vi "Find Center.vi"(5 "Position":i32, 7 "Tray Number":dbl format="%#_13g", 8 "Assembly Type":string, 9 "XYZTheta":dbl[](array[numeric]), 10 "component thickness":dbl, 11 "Gantry In":refnum<k24>) -> (0 "Pedestal Heights":dbl[][](array[numeric]), 1 "XYZTheta Centers":dbl[][](array[numeric]), 3 "Gantry Out":refnum<k24>)   [LabVIEW 2021, in "Assembly Tray.lvclass"]
uses:
  Assembly Tray.lvclass
  Find Tray.ctl
  Controller/Camera/Machine Vision.ctl
  C:/Program Files (x86)/Aerotech/A3200/LabVIEW/2010/Bin/Aerotech.A3200.dll
  Program Files (x86)/Aerotech/A3200/LabVIEW/2010/Bin/Aerotech.A3200.dll
  Controller/Camera/Image processing.ctl
  Controller/Camera/Camera settings.ctl
  <vilib>/Utility/file.llb/Read Delimited Spreadsheet (DBL).vi
  Controller/Camera/Camera.lvclass
  Controller/Motion/A3200/A3200.lvclass
  Controller/Motion/Motion.lvclass
  <vilib>/vision/NI_Vision_Development_Module.lvlib
panel:
  out "Global Report.Standard Variation":sgl
  in  "BP check":bool
  out "Program Done?":bool
  out "Manual Mode?":bool
  in  "Enter Manual Mode":bool
  out "error out":errorcluster
  out "Radius (Real-World)":dbl
  out "Match found?":bool
  out "Distance as expected?":bool
  in  "Auto Submit":bool
  out "Instructions":string="Use the joystick to match the pattern recognition until a red circle appears.\nUse Z controls to focus if needed."
  out "resulting string":string
  out "Current Z High Speed":dbl
  out "Current XY High Speed":dbl
  out "current Z low speed":dbl
  out "current XY speed":dbl
  in  "Z high":dbl=12.5
  in  "XY high":dbl=50.0
  in  "Z low":dbl=0.05
  in  "XY low":dbl=0.1
  out "Low Speed":bool
  out "X":bool
  out "Y":bool
  out "Z":bool
  out "High Speed":bool
  out "Move by":dbl[](array[numeric])
  in  "Autofiducial (Beta)":bool
  out "maximum is best focus":dbl
  in  "Focus":bool
  in  "Camera settings":T1={"Gamma"=1.6, "Gain"=0, "Sharpness"=0, "Contrast"=0.0, "Exposure"=0.0078125} {"Exposure" min=0.000244140625 max=0.5 scale=0.0002..0.5; "Contrast" min=0.0 max=1.0 scale=0.001..1.0; "Sharpness" min=0 max=2 step=1 scale=0.0..2.0; "Gain" min=0 max=100 step=1 scale=0.1..100.0; "Gamma" min=0.01 max=10.0 scale=0.01..10.0}
  in  "Image processing":T2={"Brightness"=128.0, "Contrast"=45.0, "Gamma"=1.0471123} {"Brightness" scale=0.0..400.0; "Contrast" scale=0.0..90.0; "Gamma" scale=0.005..5.0}
  in  "Override camera presets":bool
  out "Both fiducials recorded":bool
  in  "Machine Vision":T3
  out "Right Fiducial":dbl[](array[numeric]) format="%.6g"
  out "Left Fiducial":dbl[](array[numeric]) format="%.6g"
  out "Gantry":dbl[](array[numeric]) format="%.6g"
  out "Sum":dbl[](array[numeric]) format="%.6g"
  out "Camera":dbl[](array[numeric]) format="%.6g"
  in  "Carrier Tray":T4
  out "Image":T5(plugin-control)
  out "Center":dbl[](array[numeric]) format="%.6g"
  in  "Position Number":i16=1
  in  "Go to Center":bool
  in  "Calculate":bool
  in  "Record Top Right":bool
  in  "Record Top Left":bool
  in  "Go to Top Right Fiducial":bool
  in  "Go to Top Left Fiducial":bool
  in  "Joystick":bool
  in  "Stop":bool
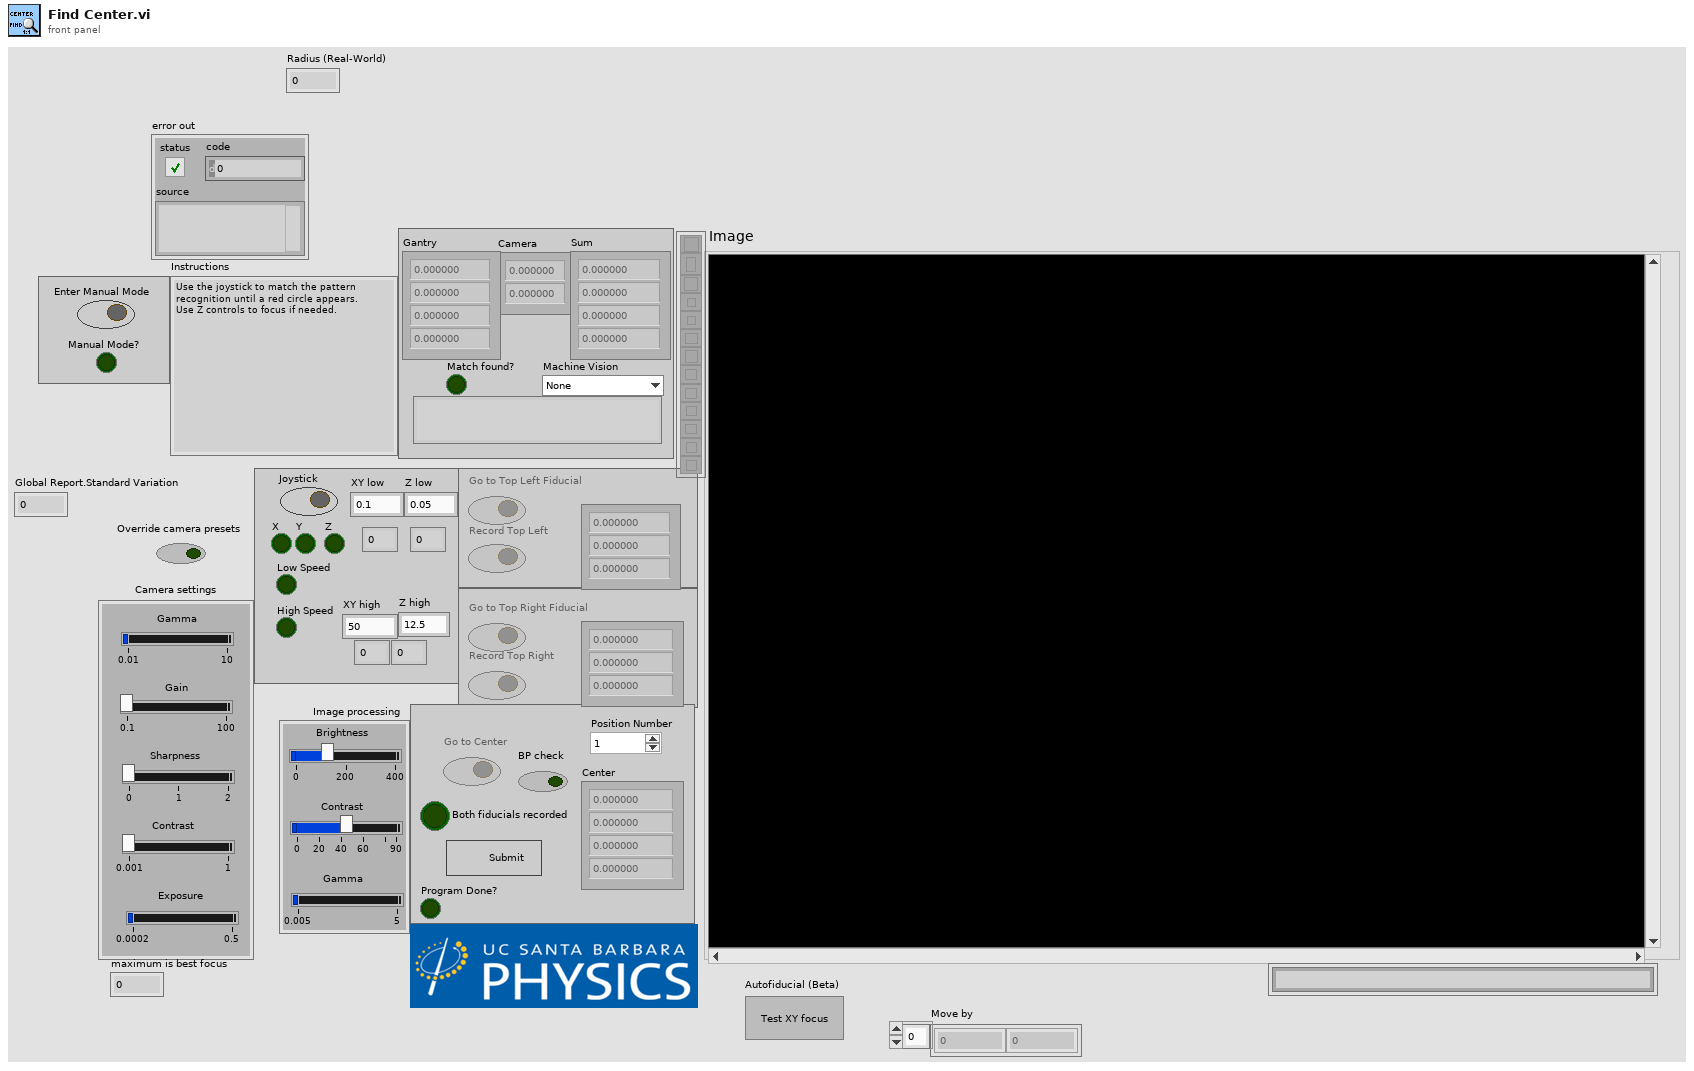
[diagram p1: front panel]
types:
  T1 = typedef "Camera.lvclass/Camera settings.ctl" = cluster{"Gamma":dbl, "Gain":i64, "Sharpness":i64, "Contrast":dbl, "Exposure":dbl}
  T2 = typedef "Camera.lvclass/Image processing.ctl" = cluster{"Brightness":sgl, "Contrast":sgl, "Gamma":sgl}
  T3 = typedef "Camera.lvclass/Machine Vision.ctl" = enum16{"None", "Assembly Tray Circle", "Assembly Tray Fiducial", "Partial Hexaboard", "sensor edge init", "HB edge init", "sensor edge pos1", "sensor edge pos2", "HB edge pos1", "HB edge pos2", "Sensor CH1-2", "HB CH1", "HB CH2", "V3 Sensor Circle", "Hexaboard Circle", "sensor CH1 check", "HB CH1 check ", "sensor ID"}
  T4 = typedef "Assembly Tray.lvclass/Find Tray.ctl" = cluster{"Gantry Fiducials":dbl[], "Relative Coordinates":dbl[][], "Camera Fiducials":dbl[][], "XYZTheta Centers":dbl[][], "Workspace Center":dbl[], "Syringe Relative Coordinates":dbl[], "Gantry Region":dbl, "Fiducials":path, "New Fiducials":dbl[][], "Past Fiducials":dbl[][], "XYZTheta":dbl[], "Pedestal Heights":dbl[][], "Assembly Type":string, "Tray Number":string, "Position":i32, "Protomodule?":bool, "avg value count":dbl[], "Previous Avgs":dbl[][], "Offset pins":dbl[][]}
  T5 = typedef "IMAQ Image.ctl" = refnum<image>
  T6 = cluster{"Average Strength":dbl, "Radius (Real-World)":dbl, "Match found?":bool, "initial angle":sgl, "Global Report":cluster{"Mean Value":sgl, "Standard Variation":sgl, "Minimal Value":sgl, "Maximal Value":sgl, "Area (calibrated)":sgl, "Area (pixels)":u32, "%":sgl, "Calibration Valid":bool}}
  T7 = enum8{"Enabled", "Disabled", "Disabled and Grayed Out"}
  T8 = typedef "File Paths.ctl" = cluster{"Glue Pattern Folder":path, "Carrier Tray Folder":path, "Pick Up Tool Fixture Folder":path, "Components Folder":path, "Bellows Tool Offset.txt":path, "Pick Up Tool Offset.txt":path, "Dispense Tip Offset.txt":path, "Log Files":path, "Gantry Assembly Map.txt":path, "Syringe and offset map.txt":path, "Controllers Folder":path, "Local dbase config":path}
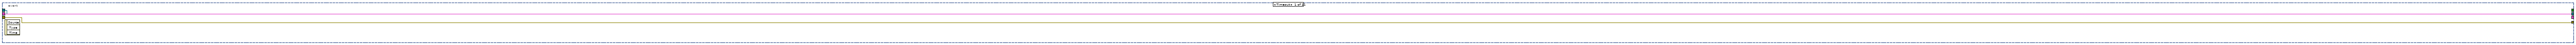
[diagram p3: hidden frame]
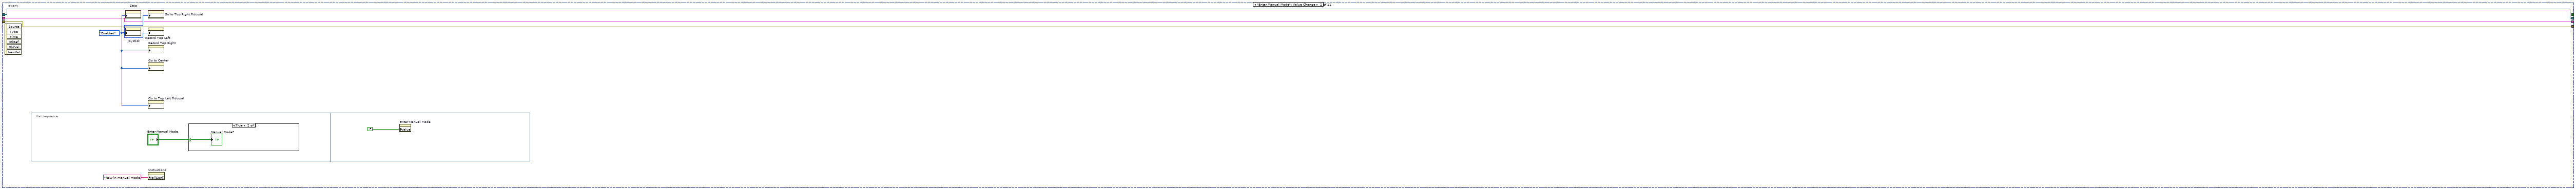
[diagram p4: hidden frame]
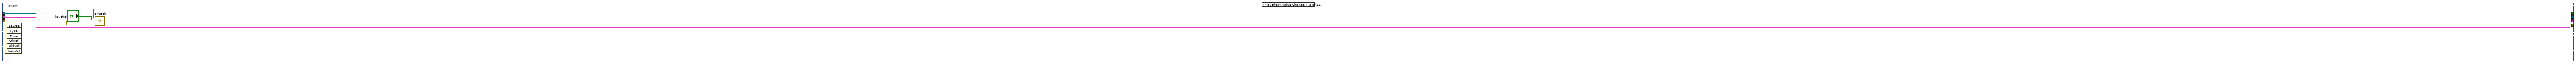
[diagram p6: hidden frame]
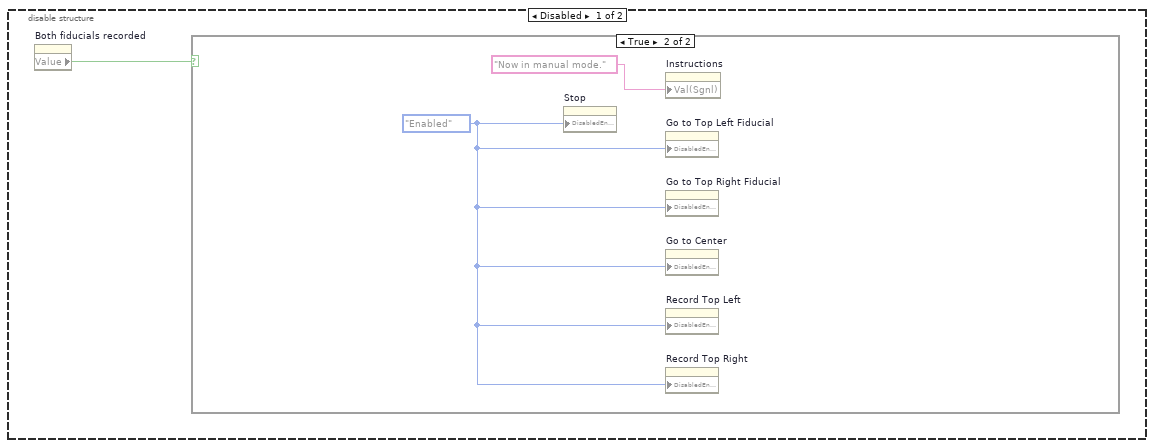
[diagram p7: hidden frame]
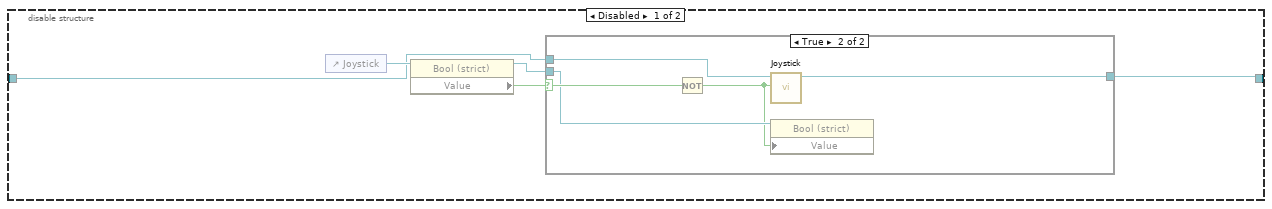
[diagram p9: hidden frame]
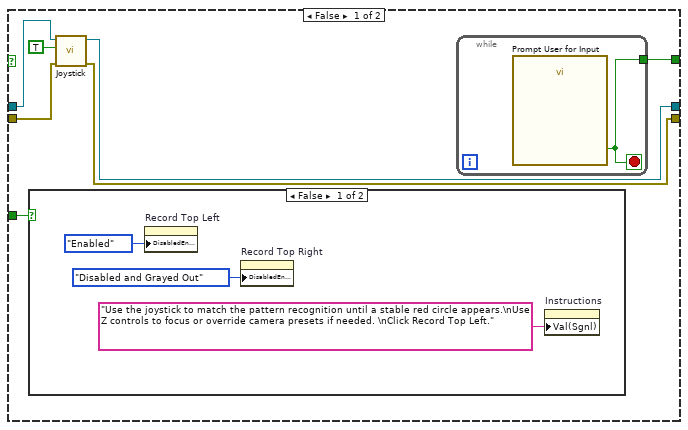
[diagram p12: hidden frame]
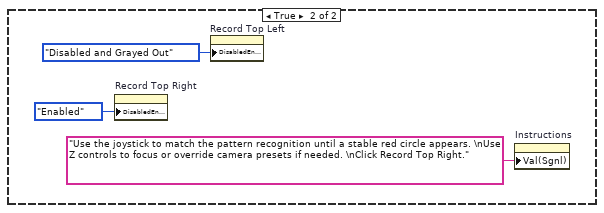
[diagram p13: hidden frame]
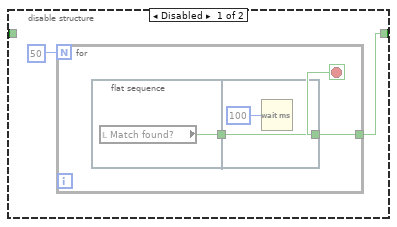
[diagram p19: hidden frame]
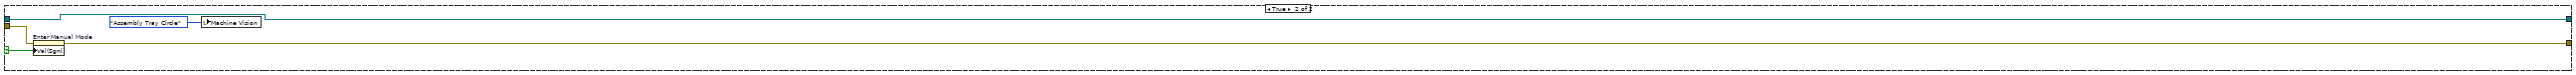
[diagram p20: hidden frame]
diagram:
  n1 = flat-sequence {
    tunnel: [w17] -> w9
    tunnel: ["Gantry In"] -> w8
    tunnel: [w16] -> w7
    tunnel: [w14] -> w4
    tunnel: [w29] -> w5
    tunnel: w9 -> [w29]
    tunnel: [w27] -> w2
    tunnel: w8 -> [w27]
    tunnel: w7 -> [w26]
    tunnel: [w26] -> w6
    tunnel: [w25] -> w1
    tunnel: w4 -> [w24]
    frame #0 {
      n2 = Decrement(x="Position") -> (x-1=w21:i32)
      n3 = call "Find Center Setup.vi"("XYZTheta"="XYZTheta", "Assembly Type"="Assembly Type", "Position"=w21, "Tray Number"="Tray Number", "Carrier Tray"="Carrier Tray") -> ("Assembly Tray Out"=w17:T4)  [unwired: 6 in]
      n4 = call "Get Camera Object.vi"() -> ("error out"=w14:errorcluster, "Camera out"=w16:refnum<class "Camera.lvclass">)  [unwired: 10 in]
    }
    frame #1 {
      n5 = control-ref of="This VI"() -> (w28:refnum<vi>)
      n6 = invoke class="VI" method="Default Vals.Reinit All"(reference=w28, error in=w24) -> (error out=w25:errorcluster)  [unwired: 1 in, 2 out]
    }
  }
  n7 = while {
    shift-right: [w36] -> _
    shift-left: w6 -> [w37]
    tunnel: w2 -> [w34]
    shift-right: [w33] -> _
    shift-left: _ -> [_]
    shift-right: [w31] -> _
    shift-left: w1 -> [w32]
    i -> [w35]
    stop <- w30 stop-if-true
    n8 = flat-sequence {
      tunnel: [w58] -> w36
      tunnel: w34 -> [w44]
      tunnel: [w43] -> w33
      tunnel: w32 -> [w42]
      tunnel: [w41] -> w31
      tunnel: w37 -> [w61]
      tunnel: w35 -> [w56]
      tunnel: [w39] -> w30
      frame #0 {
        n9 = in-place {
          in-place-border: w44 -> [w88]
          in-place-border: [w69] -> w47
          in-place-border: w42 -> [w64]
          in-place-border: [w62] -> w48
          # "Joystck Status"
          n10 = call "Get Joytick Status.vi"("error in (no error)"=w64, "Gantry In"=w88) -> ("error out"=w63:errorcluster, "JoystickLowSpeedActive"=w82:bool, "Joystick Status"=w84:bool[], "Gantry Out"=w70:refnum<k24>, "High Speeds"=w66:dbl[], "Low Speeds"=w65:dbl[])  [unwired: 4 in]
          n11 = Build Array("XY low", "XY low", "XY low", "Z low") -> (w68:dbl[])
          n12 = Build Array("XY high", "XY high", "XY high", "Z high") -> (w67:dbl[])
          n13 = call "Set Joystick Speed.vi"("error in (no error)"=w63, "High Speed Inputs"=w67, "Low Speed Inputs"=w68, "Gantry"=w70) -> ("error out"=w62:errorcluster, "Controller Out"=w69:refnum<k24>)  [unwired: 6 in]
          n14 = Or Array Elements(Boolean array=w84) -> (logical OR=w80:bool)
          n15 = Not(x=w82) -> (.not. x?=w81:bool)
          n16 = Index Array(array=w66) -> (element #1=→"Current XY High Speed":dbl, element #3=→"Current Z High Speed":dbl)  [unwired: 3 in, 1 out]
          n17 = Index Array(array=w65) -> (element #1=→"current XY speed":dbl, element #3=→"current Z low speed":dbl)  [unwired: 3 in, 1 out]
          n18 = Index Array(array=w84) -> (element #1=→"X":bool, element #2=→"Y":bool, element #3=→"Z":bool)  [unwired: 3 in]
          n19 = And(x=w80, y=w82) -> (x .and. y?=→"Low Speed":bool)
          n20 = And(x=w81, y=w80) -> (x .and. y?=→"High Speed":bool)
        }
        n21 = Equal To 0?(x=w56) -> (x = 0?=w55:bool)
        n22 = local read "Program Done?"() -> (w39:bool)
        n23 = call "Camera.vi"("Camera in"=w61, "Stop"=w39, "BCG Image Processing"="Image processing", "Machine Vision"="Machine Vision", "Camera settings"="Camera settings", "Loop 0"=w55, "Override presets"="Override camera presets") -> ("Camera out"=w58:refnum<class "Camera.lvclass">, "output cluster"=w54:T6, "Image"=→"Image":T5, "Camera"=w40:dbl[])  [unwired: 5 in, 4 out]
        "Camera" <- w40
        n24 = call "Get Current Position.vi"("error in (no error)"=w48, "Gantry In"=w47) -> ("error out"=w41:errorcluster, "XYZTheta Out"=w46:dbl[], "Gantry Out"=w43:refnum<k24>)  [unwired: 7 in]
        "Gantry" <- w46
        n25 = Unbundle By Name(w54) -> ("Average Strength"=→"maximum is best focus":dbl, "Radius (Real-World)"=→"Radius (Real-World)":dbl, "Match found?"=→"Match found?":bool, "Global Report.Standard Variation"=w38:sgl)
        "Global Report.Standard Variation" <- w38
        n26 = shared-variable ".\\Assembly Tray.lvclass\\BP Standard Variation"(w38) -> ()  [unwired: 1 in, 1 out]
        n27 = Add(x=w46, y=w40) -> (x+y=→"Sum":dbl[])
      }
    }
  }
  n28 = while {
    shift-right: [w98] -> w13
    shift-left: w5 -> [w99]
    shift-right: [w95] -> w11
    shift-left: w2 -> [w96]
    tunnel: w5 -> [w91]
    shift-right: [w89] -> w3
    shift-left: w1 -> [w90]
    i -> [w94]
    stop <- w97 stop-if-true
    n29 = event shown="[3] \"Go to Top Left Fiducial\", \"Go to Top Right Fiducial\": Value Change" {
      selector: _ -> [_ _ _ _ _ _ _ _ _ _ _]
      dyn-events: _ -> [_ _ _ _ _ _ _ _ _ _ _]
      timeout: _ -> [_ _ _ _ _ _ _ _ _ _ _]
      tunnel: [w111 w114 w125 w143 w366 w425 w563 w759 w837 w857 w930] -> w98
      tunnel: w99 -> [w111 w114 w125 w143 w362 w425 w564 w759 w838 w857 w930]
      tunnel: [_ _ _ _ _ _ _ _ _ w858 _] -> w97
      tunnel: w96 -> [w110 w115 w124 w142 w361 w424 w569 w769 w835 w861 w932]
      tunnel: [w110 w115 w122 w141 w360 w423 w569 w762 w832 w860 w933] -> w95
      tunnel: [w109 w113 w120 w132 w355 w419 w557 w763 w829 w865 w928] -> w89
      tunnel: w90 -> [w109 w113 w121 w133 w357 w418 w560 w768 w829 w862 w929]
      event Timeout {
        n30 = event-data() -> ()  [unwired: 1 in, 3 out]
      }
      event "Enter Manual Mode": Value Change {
        w116 = T7."Enabled" ("Disabled")
        n31 = event-data() -> ()  [unwired: 1 in, 6 out]
        n32 = flat-sequence {
          frame #0 {
            n33 = case shown="True" "Enter Manual Mode" {
              selector: "Enter Manual Mode" -> [_ w118]
              frame False {
              }
              frame True {
                "Manual Mode?" <- w118
              }
            }
          }
          frame #1 {
            n34 = property on="Enter Manual Mode" class="Bool (strict)"("Value"=FALSE ("Enter Manual Mode")) -> ()  [unwired: 2 in, 2 out]
          }
        }
        n35 = property on="Stop" class="Bool"("DisabledEnum"=w116) -> ()  [unwired: 2 in, 2 out]
        n36 = property on="Joystick" class="Bool (strict)"("DisabledEnum"=w116) -> ()  [unwired: 2 in, 2 out]
        n37 = property on="Go to Top Right Fiducial" class="Bool (strict)"("DisabledEnum"=w116) -> ()  [unwired: 2 in, 2 out]
        n38 = property on="Record Top Left" class="Bool (strict)"("DisabledEnum"=w116) -> ()  [unwired: 2 in, 2 out]
        n39 = property on="Record Top Right" class="Bool (strict)"("DisabledEnum"=w116) -> ()  [unwired: 2 in, 2 out]
        n40 = property on="Go to Center" class="Bool"("DisabledEnum"=w116) -> ()  [unwired: 2 in, 2 out]
        n41 = property on="Go to Top Left Fiducial" class="Bool (strict)"("DisabledEnum"=w116) -> ()  [unwired: 2 in, 2 out]
        n42 = property on="Instructions" class="Str"("Val(Sgnl)"="Now in manual mode." ("Value (Signaling)")) -> ()  [unwired: 2 in, 2 out]
      }
      event "Joystick": Value Change {
        n43 = event-data() -> ()  [unwired: 1 in, 6 out]
        n44 = call "Joystick.vi"("error in (no error)"=w121, "Joystick"="Joystick", "Gantry In"=w124) -> ("error out"=w120:errorcluster, "Gantry Out"=w122:refnum<k24>)  [unwired: 7 in]
      }
      event "Go to Top Left Fiducial", "Go to Top Right Fiducial": Value Change {
        n45 = event-data() -> ()  [unwired: 1 in, 6 out]
        n46 = disable-structure shown="Enabled" {
          frame Disabled {
            n47 = property on="Both fiducials recorded" class="Bool (strict)"() -> ("Value"=w144:bool)  [unwired: 2 in, 2 out]
            n48 = case shown="True" w144 {
              frame False {
              }
              frame True {
                w145 = T7."Enabled" ("Disabled")
                n49 = property on="Stop" class="Bool"("DisabledEnum"=w145) -> ()  [unwired: 2 in, 2 out]
                n50 = property on="Instructions" class="Str"("Val(Sgnl)"="Now in manual mode." ("Value (Signaling)")) -> ()  [unwired: 2 in, 2 out]
                n51 = property on="Go to Top Left Fiducial" class="Bool (strict)"("DisabledEnum"=w145) -> ()  [unwired: 2 in, 2 out]
                n52 = property on="Go to Top Right Fiducial" class="Bool (strict)"("DisabledEnum"=w145) -> ()  [unwired: 2 in, 2 out]
                n53 = property on="Go to Center" class="Bool"("DisabledEnum"=w145) -> ()  [unwired: 2 in, 2 out]
                n54 = property on="Record Top Left" class="Bool (strict)"("DisabledEnum"=w145) -> ()  [unwired: 2 in, 2 out]
                n55 = property on="Record Top Right" class="Bool (strict)"("DisabledEnum"=w145) -> ()  [unwired: 2 in, 2 out]
              }
            }
          }
          frame Enabled {
          }
        }
        n56 = disable-structure shown="Enabled" {
          disable-tunnel: w142 -> [w149 w158]
          disable-tunnel: [w147 w158] -> w140
          frame Disabled {
            n57 = control-ref of="Joystick"() -> (w151:refnum<vi>)
            n58 = property class="Bool (strict)"(reference=w151) -> (reference out=w148:refnum<vi>, "Value"=w150:bool)  [unwired: 1 in, 1 out]
            n59 = case shown="True" w150 {
              selector: w150 -> [_ w157]
              tunnel: w149 -> [w152 w155]
              tunnel: [w152 w154] -> w147
              tunnel: w148 -> [_ w156]
              frame False {
              }
              frame True {
                n60 = Not(x=w157) -> (.not. x?=w153:bool)
                n61 = call "Joystick.vi"("Joystick"=w153, "Gantry In"=w155) -> ("Gantry Out"=w154:refnum<k24>)  [unwired: 8 in, 1 out]
                n62 = property class="Bool (strict)"(reference=w156, "Value"=w153) -> ()  [unwired: 1 in, 2 out]
              }
            }
          }
          frame Enabled {
          }
        }
        n63 = Unbundle By Name "Unbundle By Name"(w143) -> ("Gantry Fiducials"=w135:dbl[])
        n64 = flat-sequence {
          tunnel: w135 -> [w160]
          tunnel: w140 -> [w161]
          tunnel: [w161] -> w131
          tunnel: [w160] -> w129
          tunnel: ["Go to Top Right Fiducial"] -> w127
          tunnel: ["Go to Top Right Fiducial"] -> w134
          tunnel: w131 -> [w165]
          tunnel: [w165] -> w130
          tunnel: w129 -> [w164]
          tunnel: [w164] -> w128
          tunnel: w127 -> [w163]
          tunnel: [w163] -> w126
          tunnel: [w183] -> w139
          tunnel: [w179] -> w136
          tunnel: w130 -> [w177]
          tunnel: w128 -> [w174]
          tunnel: w126 -> [w171]
          tunnel: w133 -> [w167]
          tunnel: w139 -> [w185]
          tunnel: [w185] -> w138
          tunnel: [w184] -> w137
          tunnel: w136 -> [w184]
          tunnel: [w188] -> w141
          tunnel: [w187] -> w132
          tunnel: w137 -> [w190]
          tunnel: w134 -> [w191]
          tunnel: w138 -> [w192]
          frame #0 {
          }
          frame #1 {
            w162 = FALSE ("Go to Top Right Fiducial")
            n65 = property on="Go to Top Left Fiducial" class="Bool (strict)"("Value"=w162) -> ()  [unwired: 2 in, 2 out]
            n66 = property on="Go to Top Right Fiducial" class="Bool (strict)"("Value"=w162) -> ()  [unwired: 2 in, 2 out]
          }
          frame #2 {
            w180 = T7."Disabled and Grayed Out" ("Disabled")
            n67 = Select(t=3, s=w171, f=0) -> (s? t:f=w169:i32)
            n68 = call "Joystick.vi"("error in (no error)"=w167, "Joystick"=FALSE, "Gantry In"=w177) -> ("error out"=w175:errorcluster, "Gantry Out"=w178:refnum<k24>)  [unwired: 7 in]
            n69 = Array Subset "Array Subset"(array=w174, index=w169, length=3) -> (w173:dbl[])
            n70 = property on="Instructions" class="Str"("Val(Sgnl)"="Wait for movement to stop." ("Value (Signaling)")) -> ()  [unwired: 2 in, 2 out]
            n71 = property on="Go to Center" class="Bool"("DisabledEnum"=w180) -> ()  [unwired: 2 in, 2 out]
            n72 = property on="Stop" class="Bool"("DisabledEnum"=w180) -> ()  [unwired: 2 in, 2 out]
            n73 = property on="Record Top Right" class="Bool (strict)"("DisabledEnum"=w180) -> ()  [unwired: 2 in, 2 out]
            n74 = property on="Go to Top Right Fiducial" class="Bool (strict)"("DisabledEnum"=w180) -> ()  [unwired: 2 in, 2 out]
            n75 = property on="Go to Top Left Fiducial" class="Bool (strict)"("DisabledEnum"=w180) -> ()  [unwired: 2 in, 2 out]
            n76 = property on="Record Top Left" class="Bool (strict)"("DisabledEnum"=w180) -> ()  [unwired: 2 in, 2 out]
            n77 = local write "Machine Vision"(Machine_Vision."Assembly Tray Fiducial" ("Machine Vision")) -> ()
            n78 = call "ClearXYZTheta Go.vi"("error in (no error)"=w175, "Speed"=300.0, "XYZTheta In"=w173, "Gantry In"=w178) -> ("error out"=w179:errorcluster, "Gantry Out"=w183:refnum<k24>)  [unwired: 5 in, 1 out]
          }
          frame #3 {
            n79 = disable-structure shown="Enabled" {
              frame Enabled {
                n80 = Wait (ms)(milliseconds to wait=u32 1000) -> ()  [unwired: 1 out]
              }
              frame Disabled {
              }
            }
          }
          frame #4 {
            n81 = local read "Manual Mode?"() -> (w189:bool)
            n82 = case shown="False" w189 {
              selector: w189 -> [_ w352]
              tunnel: w192 -> [w214 w353]
              tunnel: [w194 w353] -> w188
              tunnel: w191 -> [w195 _]
              tunnel: w190 -> [w213 w351]
              tunnel: [w193 w350] -> w187
              frame False {
                n83 = flat-sequence {
                  tunnel: w214 -> [w239]
                  tunnel: w213 -> [w237]
                  tunnel: [w238] -> w212
                  tunnel: [w236] -> w211
                  tunnel: [w235] -> w210
                  tunnel: [w234] -> w209
                  tunnel: w212 -> [w299]
                  tunnel: w211 -> [w298]
                  tunnel: w210 -> [w297]
                  tunnel: w209 -> [w296]
                  tunnel: [w299] -> w208
                  tunnel: [w298] -> w206
                  tunnel: [w297] -> w204
                  tunnel: [w296] -> w202
                  tunnel: w208 -> [w303]
                  tunnel: [w303] -> w207
                  tunnel: w206 -> [w302]
                  tunnel: [w302] -> w205
                  tunnel: w204 -> [w301]
                  tunnel: [w301] -> w203
                  tunnel: w202 -> [w300]
                  tunnel: [w300] -> w201
                  tunnel: w207 -> [w311]
                  tunnel: w205 -> [w310]
                  tunnel: w203 -> [w306]
                  tunnel: w201 -> [w309]
                  tunnel: [w308] -> w199
                  tunnel: [w307] -> w200
                  tunnel: [w305] -> w196
                  frame #0 {
                    n84 = for {
                      N: 50 -> [_]
                      tunnel: [w242] -> w240
                      tunnel: [w241] -> w232
                      stop <- w242 stop-if-true
                      n85 = flat-sequence {
                        tunnel: [w245] -> w243
                        tunnel: [w244] -> w241
                        tunnel: [w247] -> w242
                        tunnel: w243 -> [w247]
                        frame #0 {
                          n86 = local read "Match found?"() -> (w245:bool)
                          n87 = local read "Camera"() -> (w244:dbl[])
                        }
                        frame #1 {
                          n88 = Wait (ms)(milliseconds to wait=u32 100) -> ()  [unwired: 1 out]
                        }
                      }
                    }
                    n89 = case shown="False" w240 {
                      selector: w240 -> [_ w292]
                      tunnel: w239 -> [w251 w294]
                      tunnel: [w253 w294] -> w238
                      tunnel: w237 -> [w250 w293]
                      tunnel: [w252 w293] -> w236
                      tunnel: [w249 w292] -> w235
                      tunnel: [w248 w291] -> w234
                      tunnel: w232 -> [_ w291]
                      frame False {
                        n90 = flat-sequence {
                          tunnel: [w265] -> w253
                          tunnel: [w264] -> w252
                          tunnel: w251 -> [w263]
                          tunnel: w250 -> [w262]
                          tunnel: [w257] -> w249
                          tunnel: [w254] -> w248
                          frame #0 {
                            n91 = call "Base File Path.vi"() -> ("Paths Out"=w259:T8)  [unwired: 11 in]
                            n92 = Unbundle By Name(w259) -> ("Controllers Folder"=w260:path)
                            n93 = String To Path(string="Scan.txt") -> (path=w261:path)
                            n94 = Build Path(base path=w260, name or relative path=w261) -> (appended path=w256:path)
                            n95 = call-poly <vilib>:"Read Delimited Spreadsheet.vi"("file path (dialog if empty)"=w256) -> ("all rows"=w255:dbl[][])  [unwired: 9 in, 5 out]
                            n96 = for {
                              shift-right: [w275] -> w265
                              shift-left: w263 -> [w276]
                              tunnel: w255 -> [w274] mode=indexing
                              shift-right: [w272] -> w264
                              shift-left: w262 -> [w273]
                              tunnel: [w267] -> w257
                              tunnel: [w266] -> w254
                              stop <- w267 stop-if-true
                              n97 = flat-sequence {
                                tunnel: w276 -> [w283]
                                tunnel: w274 -> [w281]
                                tunnel: w273 -> [w279]
                                tunnel: [w282] -> w271
                                tunnel: [w278] -> w270
                                tunnel: w271 -> [w284]
                                tunnel: w270 -> [w285]
                                tunnel: [w284] -> w269
                                tunnel: [w285] -> w268
                                tunnel: [w289] -> w272
                                tunnel: [w290] -> w275
                                tunnel: w269 -> [w290]
                                tunnel: w268 -> [w289]
                                tunnel: [w288] -> w267
                                tunnel: [w287] -> w266
                                frame #0 {
                                n98 = call "XY Go.vi"("Increment?"=TRUE, "error in (no error)"=w279, "Speed"=0.1, "XY In"=w281, "Gantry In"=w283) -> ("error out"=w278:errorcluster, "Gantry Out"=w282:refnum<k24>)  [unwired: 4 in, 1 out]
                                }
                                frame #1 {
                                n99 = disable-structure shown="Enabled" {
                                disable-tunnel: w284 -> [_ _]
                                frame Enabled {
                                n100 = Wait (ms)(milliseconds to wait=u32 500) -> ()  [unwired: 1 out]
                                }
                                frame Disabled {
                                }
                                }
                                }
                                frame #2 {
                                n101 = local read "Match found?"() -> (w288:bool)
                                n102 = local read "Camera"() -> (w287:dbl[])
                                }
                              }
                            }
                          }
                        }
                      }
                      frame True {
                      }
                    }
                  }
                  frame #1 {
                    n103 = local write "Machine Vision"(Machine_Vision."Assembly Tray Circle" ("Machine Vision")) -> ()
                  }
                  frame #2 {
                    n104 = disable-structure shown="Enabled" {
                      frame Enabled {
                        n105 = Wait (ms)(milliseconds to wait=u32 1000) -> ()  [unwired: 1 out]
                      }
                      frame Disabled {
                      }
                    }
                  }
                  frame #3 {
                    n106 = case shown="True" w306 {
                      selector: w306 -> [w312 w315]
                      tunnel: w311 -> [w314 w325]
                      tunnel: [w314 w324] -> w308
                      tunnel: w310 -> [w313 w323]
                      tunnel: [w313 w322] -> w307
                      tunnel: w309 -> [_ w321]
                      tunnel: [w312 w316] -> w305
                      frame False {
                      }
                      frame True {
                        n107 = flat-sequence {
                          tunnel: w325 -> [w333]
                          tunnel: w323 -> [w331]
                          tunnel: w321 -> [w326]
                          tunnel: [w332] -> w320
                          tunnel: [w330] -> w319
                          tunnel: w320 -> [w335]
                          tunnel: w319 -> [w334]
                          tunnel: [w335] -> w318
                          tunnel: [w334] -> w317
                          tunnel: [w339] -> w322
                          tunnel: [w340] -> w324
                          tunnel: w318 -> [w340]
                          tunnel: w317 -> [w339]
                          tunnel: [w338] -> w316
                          tunnel: w315 -> [w337]
                          frame #0 {
                            n108 = call "XY Go.vi"("Increment?"=TRUE, "error in (no error)"=w331, "Speed"=5.0, "XY In"=w326, "Gantry In"=w333) -> ("error out"=w330:errorcluster, "Gantry Out"=w332:refnum<k24>)  [unwired: 4 in, 1 out]
                            n109 = property on="Instructions" class="Str"("Val(Sgnl)"="Fiducial found." ("Value (Signaling)")) -> ()  [unwired: 2 in, 2 out]
                          }
                          frame #1 {
                            n110 = disable-structure shown="Enabled" {
                              frame Enabled {
                                n111 = Wait (ms)(milliseconds to wait=u32 1000) -> ()  [unwired: 1 out]
                              }
                              frame Disabled {
                              }
                            }
                          }
                          frame #2 {
                            n112 = disable-structure shown="Enabled" {
                              disable-tunnel: [w342 w348] -> w338
                              disable-tunnel: w337 -> [_ w348]
                              frame Disabled {
                                n113 = for {
                                N: 50 -> [_]
                                tunnel: [w343] -> w342
                                stop <- w343 stop-if-true
                                n114 = flat-sequence {
                                tunnel: [w345] -> w344
                                tunnel: [w347] -> w343
                                tunnel: w344 -> [w347]
                                frame #0 {
                                n115 = local read "Match found?"() -> (w345:bool)
                                }
                                frame #1 {
                                n116 = Wait (ms)(milliseconds to wait=u32 100) -> ()  [unwired: 1 out]
                                }
                                }
                                }
                              }
                              frame Enabled {
                              }
                            }
                          }
                        }
                      }
                    }
                  }
                }
                n117 = case shown="True" w196 {
                  selector: w196 -> [_ w231]
                  tunnel: [w216 w231] -> w198
                  tunnel: w199 -> [w220 w230]
                  tunnel: [w219 w230] -> w194
                  tunnel: w200 -> [w218 w229]
                  tunnel: [w217 w229] -> w197
                  tunnel: w195 -> [w215 _]
                  frame False {
                    n118 = case shown="False" w215 {
                      frame False {
                        n119 = property on="Record Top Left" class="Bool (strict)"("DisabledEnum"=T7."Enabled" ("Disabled")) -> ()  [unwired: 2 in, 2 out]
                        n120 = property on="Record Top Right" class="Bool (strict)"("DisabledEnum"=T7."Disabled and Grayed Out" ("Disabled")) -> ()  [unwired: 2 in, 2 out]
                        n121 = property on="Instructions" class="Str"("Val(Sgnl)"="Use the joystick to match the pattern recognition until a stable red circle appears.\nUse Z controls to focus or override camera presets if needed. \nClick Record Top Left.") -> ()  [unwired: 2 in, 2 out]
                      }
                      frame True {
                        n122 = property on="Record Top Right" class="Bool (strict)"("DisabledEnum"=T7."Enabled" ("Disabled")) -> ()  [unwired: 2 in, 2 out]
                        n123 = property on="Record Top Left" class="Bool (strict)"("DisabledEnum"=T7."Disabled and Grayed Out" ("Disabled")) -> ()  [unwired: 2 in, 2 out]
                        n124 = property on="Instructions" class="Str"("Val(Sgnl)"="Use the joystick to match the pattern recognition until a stable red circle appears. \nUse Z controls to focus or override camera presets if needed. \nClick Record Top Right.") -> ()  [unwired: 2 in, 2 out]
                      }
                    }
                    n125 = call "Joystick.vi"("error in (no error)"=w218, "Joystick"=TRUE, "Gantry In"=w220) -> ("error out"=w217:errorcluster, "Gantry Out"=w219:refnum<k24>)  [unwired: 7 in]
                    n126 = while {
                      tunnel: [w222] -> w216
                      stop <- w222 stop-if-true
                      n127 = call "Prompt User for Input"() -> ("Target line up?"=w222:bool)  [unwired: 17 in, 2 out]
                    }
                  }
                  frame True {
                  }
                }
                n128 = property on="Focus" class="Bool (strict)"(error in=w197, "Val(Sgnl)"=w198) -> (error out=w193:errorcluster)  [unwired: 1 in, 1 out]
              }
              frame True {
                n129 = property on="Enter Manual Mode" class="Bool (strict)"(error in=w351, "Val(Sgnl)"=w352) -> (error out=w350:errorcluster)  [unwired: 1 in, 1 out]
                n130 = local write "Machine Vision"(Machine_Vision."Assembly Tray Circle" ("Machine Vision")) -> ()
              }
            }
          }
        }
      }
      event "Record Top Left", "Record Top Right": Value Change {
        n131 = event-data() -> ()  [unwired: 1 in, 6 out]
        n132 = flat-sequence {
          tunnel: ["Record Top Right"] -> w354
          frame #0 {
          }
          frame #1 {
            w368 = FALSE ("Record Top Left")
            n133 = property on="Record Top Left" class="Bool (strict)"("Value"=w368) -> ()  [unwired: 2 in, 2 out]
            n134 = property on="Record Top Right" class="Bool (strict)"("Value"=w368) -> ()  [unwired: 2 in, 2 out]
          }
        }
        n135 = Boolean To (0,1)(Boolean=w354) -> (0, 1=w363:i16)
        n136 = in-place {
          in-place-border: [w387] -> w364
          in-place-border: w363 -> [w380]
          in-place-border: w361 -> [w382]
          in-place-border: [w381] -> w360
          in-place-border: w357 -> [w375]
          in-place-border: [w373] -> w356
          n137 = in-place-cluster #1(w362) -> ("Gantry Fiducials"=w384:dbl[], "Camera Fiducials"=w391:dbl[][])
          n138 = call "Get Current Position.vi"("error in (no error)"=w375, "Gantry In"=w382) -> ("error out"=w374:errorcluster, "XYZTheta Out"=w385:dbl[], "Gantry Out"=w381:refnum<k24>)  [unwired: 7 in]
          n139 = Multiply(x=w380, y=i16 3) -> (x*y=w378:i16)
          n140 = Reshape Array(w385, 3 ("dimension size")) -> (w377:dbl[])
          n141 = Replace Array Subset(array=w384, new element=w377, index=w378) -> (w383:dbl[])
          n142 = in-place {
            n143 = in-place-array #2(w377, 0, 1) -> (w399:dbl, w397:dbl)
            n144 = local read "Camera"() -> (w400:dbl[])
            n145 = Index Array(array=w400) -> (element #1=w398:dbl, element #2=w396:dbl)  [unwired: 2 in]
            n146 = Add(x=w399, y=w398) -> (x+y=w394:dbl)
            n147 = Add(x=w397, y=w396) -> (x+y=w395:dbl)
            n148 = in-place-array #2(w394, w395) -> (w376:dbl[])  [unwired: 2 out]
          }
          n149 = Reshape Array(w391, 2 ("length"), 3 ("dimension size")) -> (w390:dbl[][])
          n150 = case shown="0, Default" w380 {
            tunnel: w376 -> [w404 w416]
            tunnel: w374 -> [w403 w415]
            tunnel: [w402 w415] -> w373
            frame 0, Default {
              n151 = local read "Manual Mode?"() -> (w401:bool)
              n152 = case shown="True" w401 {
                selector: w401 -> [_ w414]
                tunnel: w403 -> [w406 w413]
                tunnel: [w405 w412] -> w402
                frame False {
                  n153 = property on="Both fiducials recorded" class="Bool (strict)"() -> ("Value"=w407:bool)  [unwired: 2 in, 2 out]
                  n154 = case shown="False" w407 {
                    tunnel: w406 -> [w409 w411]
                    tunnel: [w408 w411] -> w405
                    frame False {
                      n155 = property on="Go to Top Right Fiducial" class="Bool (strict)"(error in=w409, "Val(Sgnl)"=TRUE ("Value (Signaling)")) -> (error out=w408:errorcluster)  [unwired: 1 in, 1 out]
                    }
                    frame True {
                    }
                  }
                }
                frame True {
                  n156 = property on="Enter Manual Mode" class="Bool (strict)"(error in=w413, "Val(Sgnl)"=w414) -> (error out=w412:errorcluster)  [unwired: 1 in, 1 out]
                }
              }
              "Left Fiducial" <- w404
            }
            frame 1 {
              "Right Fiducial" <- w416
            }
          }
          n157 = Replace Array Subset(array=w390, new element=w376, index (row)=w380) -> (w387:dbl[][])  [unwired: 1 in]
          n158 = in-place-cluster #1("Gantry Fiducials"=w383, "Camera Fiducials"=w387) -> (w366:T4)
        }
        n159 = Multiply Array Elements(1:w364) -> (0:w365:dbl)
        n160 = Equal To 0?(x=w365) -> (x = 0?=w359:bool)
        n161 = Not(x=w359) -> (.not. x?=→"Both fiducials recorded":bool)
        n162 = case shown="False" w359 {
          selector: w359 -> [w371 _]
          tunnel: w356 -> [w370 w372]
          tunnel: [w369 w372] -> w355
          frame False {
            n163 = property on="Calculate" class="Bool (strict)"(error in=w370, "Val(Sgnl)"=w371) -> (error out=w369:errorcluster)  [unwired: 1 in, 1 out]
          }
          frame True {
          }
        }
      }
      event "Focus": Value Change {
        n164 = event-data() -> ()  [unwired: 1 in, 6 out]
        n165 = flat-sequence {
          tunnel: w418 -> [w428]
          tunnel: [w426] -> w417
          tunnel: w424 -> [w433]
          tunnel: [w432] -> w422
          tunnel: [w431] -> w421
          tunnel: [w430] -> w420
          tunnel: w417 -> [w429]
          tunnel: [w522] -> w423
          tunnel: w422 -> [w523]
          tunnel: w421 -> [w525]
          tunnel: w420 -> [w524]
          tunnel: [w521] -> w419
          frame #0 {
            n166 = property on="Focus" class="Bool (strict)"(error in=w428, "Value"=FALSE ("Focus")) -> (error out=w426:errorcluster)  [unwired: 1 in, 1 out]
          }
          frame #1 {
            n167 = local read "Match found?"() -> (w434:bool)
            n168 = case shown="False" w434 {
              tunnel: w433 -> [w462 w518]
              tunnel: [w450 w518] -> w432
              tunnel: [w451 w517] -> w431
              tunnel: w429 -> [w436 w517]
              tunnel: [w439 FALSE ("empty?")] -> w430
              frame False {
                n169 = property on="Instructions" class="Str"(error in=w436, "Val(Sgnl)"="Now finding best focus." ("Value (Signaling)")) -> (error out=w435:errorcluster)  [unwired: 1 in, 1 out]
                n170 = call "Joystick.vi"("error in (no error)"=w435, "Joystick"=FALSE, "Gantry In"=w462) -> ("error out"=w443:errorcluster, "Gantry Out"=w447:refnum<k24>)  [unwired: 7 in]
                n171 = call "Get Current Position.vi"("error in (no error)"=w443, "Gantry In"=w447) -> ("error out"=w445:errorcluster, "XYZTheta Out"=w444:dbl[], "Gantry Out"=w446:refnum<k24>)  [unwired: 7 in]
                n172 = call "Z Go.vi"("Increment"=TRUE, "Return Immediately"=FALSE ("Increment"), "error in (no error)"=w445, "Speed In"=1.0 ("Speed"), "Position In"=-0.1, "Gantry In"=w446) -> ("error out"=w458:errorcluster, "Gantry Out"=w461:refnum<k24>)  [unwired: 2 in, 2 out]
                n173 = for {
                  N: 20 -> [_]
                  shift-right: [w481] -> w452
                  shift-left: w461 -> [w483]
                  shift-right: [w480] -> w466
                  shift-left: dbl[][] [] -> [w473]
                  shift-right: [w477] -> w454
                  shift-left: w458 -> [w479]
                  n174 = flat-sequence {
                    tunnel: w483 -> [w486]
                    tunnel: [w486] -> w482
                    tunnel: w479 -> [w485]
                    tunnel: [w485] -> w478
                    tunnel: w482 -> [w493]
                    tunnel: w478 -> [w490]
                    tunnel: [w492] -> w476
                    tunnel: [w491] -> w475
                    tunnel: [w489] -> w474
                    tunnel: w473 -> [w487]
                    tunnel: [w509] -> w477
                    tunnel: [w515] -> w480
                    tunnel: [w510] -> w481
                    tunnel: w476 -> [w511]
                    tunnel: w475 -> [w515]
                    tunnel: w474 -> [w508]
                    frame #0 {
                      n175 = Wait (ms)(milliseconds to wait=u32 500) -> ()  [unwired: 1 out]
                    }
                    frame #1 {
                      n176 = local read "Match found?"() -> (w488:bool)
                      n177 = case shown="True" w488 {
                        tunnel: w493 -> [w495 w506]
                        tunnel: [w495 w505] -> w492
                        tunnel: [w494 w497] -> w491
                        tunnel: w490 -> [w496 w501]
                        tunnel: [w496 w500] -> w489
                        tunnel: w487 -> [w494 _]
                        frame False {
                        }
                        frame True {
                          n178 = call "Get Current Position.vi"("error in (no error)"=w501, "Gantry In"=w506) -> ("error out"=w500:errorcluster, "XYZTheta Out"=w504:dbl[], "Gantry Out"=w505:refnum<k24>)  [unwired: 7 in]
                          n179 = local read "maximum is best focus"() -> (w499:dbl)
                          n180 = Delete From Array(array=w504, index=2) -> (deleted portion=w502:dbl)  [unwired: 1 in, 1 out]
                          n181 = Build Array(w499, w502) -> (w498:dbl[])
                          n182 = Build Array(w498) -> (w497:dbl[][])
                        }
                      }
                    }
                    frame #2 {
                      n183 = call "Z Go.vi"("Increment"=TRUE, "Return Immediately"=FALSE ("Increment"), "error in (no error)"=w508, "Speed In"=1.0 ("Speed"), "Position In"=0.01, "Gantry In"=w511) -> ("error out"=w509:errorcluster, "Gantry Out"=w510:refnum<k24>)  [unwired: 2 in, 2 out]
                    }
                  }
                }
                n184 = Transpose 2D Array(2D array=w466) -> (transposed array=w465:dbl[][])
                n185 = Index Array(array=w465) -> (element #1=w440:dbl[], element #2=w464:dbl[])  [unwired: 4 in]
                n186 = Empty Array?(array=w440) -> (empty?=w439:bool)
                n187 = Array Max & Min(array=w440) -> (max index (indices)=w441:i32)  [unwired: 3 out]
                n188 = case shown="False" w439 {
                  tunnel: w464 -> [w469 _]
                  tunnel: w441 -> [w468 _]
                  tunnel: [w467 w470] -> w453
                  tunnel: w444 -> [_ w472]
                  frame False {
                    n189 = Index Array(array=w469, index=w468) -> (element=w467:dbl)
                  }
                  frame True {
                    n190 = Index Array(array=w472, index=2) -> (element=w470:dbl)
                  }
                }
                n191 = call "Z Go.vi"("Increment"=FALSE, "Return Immediately"=FALSE ("Increment"), "error in (no error)"=w454, "Speed In"=15.0 ("Speed"), "Position In"=w453, "Gantry In"=w452) -> ("error out"=w451:errorcluster, "Gantry Out"=w450:refnum<k24>)  [unwired: 2 in, 2 out]
              }
              frame True {
              }
            }
          }
          frame #2 {
            n192 = local read "Left Fiducial"() -> (w520:dbl[])
            n193 = Empty Array?(array=w520) -> (empty?=w519:bool)
            n194 = case shown="True" w524 {
              tunnel: [w528 w542] -> w522
              tunnel: w525 -> [w529 w539]
              tunnel: w523 -> [w528 w540]
              tunnel: [w527 w538] -> w521
              tunnel: w519 -> [w526 w537]
              frame False {
                n195 = case shown="False" w526 {
                  selector: w526 -> [_ w534]
                  tunnel: w529 -> [w531 w535]
                  tunnel: [w530 w533] -> w527
                  frame False {
                    n196 = property on="Record Top Right" class="Bool (strict)"(error in=w531, "Val(Sgnl)"=TRUE ("Value (Signaling)")) -> (error out=w530:errorcluster)  [unwired: 1 in, 1 out]
                  }
                  frame True {
                    n197 = property on="Record Top Left" class="Bool (strict)"(error in=w535, "Val(Sgnl)"=w534) -> (error out=w533:errorcluster)  [unwired: 1 in, 1 out]
                  }
                }
              }
              frame True {
                n198 = case shown="True" w537 {
                  frame False {
                    n199 = property on="Record Top Right" class="Bool (strict)"("DisabledEnum"=T7."Enabled" ("Disabled")) -> ()  [unwired: 2 in, 2 out]
                    n200 = property on="Record Top Left" class="Bool (strict)"("DisabledEnum"=T7."Disabled and Grayed Out" ("Disabled")) -> ()  [unwired: 2 in, 2 out]
                    n201 = property on="Instructions" class="Str"("Val(Sgnl)"="Use the joystick to match the pattern recognition until a stable red circle appears. \nUse Z controls to focus or override camera presets if needed. \nClick Record Top Right.") -> ()  [unwired: 2 in, 2 out]
                  }
                  frame True {
                    n202 = property on="Record Top Left" class="Bool (strict)"("DisabledEnum"=T7."Enabled" ("Disabled")) -> ()  [unwired: 2 in, 2 out]
                    n203 = property on="Record Top Right" class="Bool (strict)"("DisabledEnum"=T7."Disabled and Grayed Out" ("Disabled")) -> ()  [unwired: 2 in, 2 out]
                    n204 = property on="Instructions" class="Str"("Val(Sgnl)"="Use the joystick to match the pattern recognition until a stable red circle appears.\nUse Z controls to focus or override camera presets if needed. \nClick Record Top Left.") -> ()  [unwired: 2 in, 2 out]
                  }
                }
                n205 = call "Joystick.vi"("error in (no error)"=w539, "Joystick"=TRUE, "Gantry In"=w540) -> ("error out"=w538:errorcluster, "Gantry Out"=w542:refnum<k24>)  [unwired: 7 in]
                n206 = One Button Dialog(message="Warning: Focus failed. Find fiducial manually with joystick. See instructions for more information.") -> ()  [unwired: 1 in, 1 out]
              }
            }
          }
        }
      }
      event "Calculate": Value Change {
        n207 = event-data() -> ()  [unwired: 1 in, 6 out]
        n208 = disable-structure shown="Enabled" {
          frame Disabled {
            n209 = control-ref of="Position Number"() -> (w752:refnum<vi>)
            n210 = property class="DigNum (strict)"(reference=w752, "Val(Sgnl)"=i16 1 ("Value (Signaling)")) -> ()  [unwired: 1 in, 2 out]
          }
          frame Enabled {
          }
        }
        n211 = Unbundle By Name "Unbundle By Name"(w564) -> ("Camera Fiducials"=w567:dbl[][], "Relative Coordinates"=w568:dbl[][], "Assembly Type"=w562:string, "Protomodule?"=w556:bool)  [unwired: 1 out]
        n212 = case shown="\"Module HD Full\"" w562 {
          tunnel: ["Calculate_Centers" ("function name") "Calculate_Centers" ("function name") "Calculate_Centers" ("function name") "Calculate_Centers" ("function name") "Calculate_Centers_Right_Partial" ("function name") "Calculate_Centers_Right_Partial" ("function name")] -> w566
          frame "Protomodule LD Full", Default {
          }
          frame "Protomodule HD Full" {
          }
          frame "Module LD Full" {
          }
          frame "Module HD Full" {
          }
          frame "Module LD Right" {
          }
          frame "Protomodule LD Right" {
          }
        }
        n213 = property on="Calculate" class="Bool (strict)"(error in=w560, "Value"=FALSE ("Calculate")) -> (error out=w559:errorcluster)  [unwired: 1 in, 1 out]
        n214 = Build Array(w567, w568) -> (w565:dbl[][][])
        n215 = for {
          tunnel: w565 -> [w740] mode=indexing
          shift-right: [w738] -> w558
          shift-left: w559 -> [w739]
          tunnel: [w736] -> w555 mode=indexing
          n216 = Array Subset(array=w740, index (row)=0 ("index"), length (row)=2 ("length"), index (col)=0 ("index"), length (col)=2 ("length")) -> (w743:dbl[][])
          n217 = Index Array(array=w743) -> (element #1=w742:dbl[], element #2=w741:dbl[])  [unwired: 4 in]
          n218 = Array To Cluster(array=w742) -> (cluster=w746:cluster{"[0]":dbl, "[1]":dbl})
          n219 = Array To Cluster(array=w741) -> (cluster=w745:cluster{"[0]":dbl, "[1]":dbl})
          n220 = Build Array(w746, w745) -> (w744:cluster{"[0]":dbl, "[1]":dbl}[])
          n221 = call "IMAQ Point Distances"("Points"=w744, "error in (no error)"=w739) -> ("Distances"=w737:sgl[], "error out"=w738:errorcluster)  [unwired: 3 in]
          n222 = Index Array(array=w737) -> (element=w736:sgl)  [unwired: 1 in]
        }
        n223 = Index Array(array=w555) -> (element #1=w554:sgl, element #2=w553:sgl)  [unwired: 2 in]
        n224 = Subtract(x=w554, y=w553) -> (x-y=w552:sgl)
        n225 = Absolute Value(x=w552) -> (abs(x)=w551:sgl)
        n226 = Less?(x=w551, y=sgl 0.02) -> (x < y?=w549:bool)
        "Distance as expected?" <- w549
        n227 = case shown="True" w549 {
          tunnel: w568 -> [_ w591]
          tunnel: w566 -> [_ w589]
          tunnel: w567 -> [_ w588]
          tunnel: w564 -> [w573 w587]
          tunnel: [w573 w582] -> w563
          tunnel: w558 -> [w571 w581]
          tunnel: [w570 w578] -> w557
          tunnel: w556 -> [_ w577]
          frame False {
            n228 = property on="Enter Manual Mode" class="Bool (strict)"(error in=w571, "Val(Sgnl)"=TRUE ("Value (Signaling)")) -> (error out=w570:errorcluster)  [unwired: 1 in, 1 out]
            n229 = One Button Dialog(message="Error: Distance between fiducials does not match expected.\nReview fiducials manually.") -> ()  [unwired: 1 in, 1 out]
          }
          frame True {
            n230 = call "Get Python Version.vi"("error in (no error)"=w581) -> ("Python Version"=w599:string, "error out"=w600:errorcluster)  [unwired: 9 in]
            n231 = Open Python Session(python version=w599, 3:w600) -> (session out=w592:refnum<k35>, error out=w594:errorcluster)  [unwired: 1 in]
            n232 = call "Base File Path.vi"() -> ("Paths Out"=w596:T8)  [unwired: 11 in]
            n233 = Unbundle By Name(w596) -> ("Carrier Tray Folder"=w597:path)
            n234 = Build Path(base path=w597, name or relative path=path "Calculate Baseplate Center.py") -> (appended path=w598:path)
            n235 = disable-structure shown="Enabled" {
              disable-tunnel: w598 -> [w613 w624 w638 w651 _]
              disable-tunnel: [w612 w623 w637 w650 _] -> w595
              disable-tunnel: w594 -> [w611 w622 w636 w649 _]
              disable-tunnel: [w610 w621 w635 w648 _] -> w593
              disable-tunnel: w592 -> [w609 w620 w634 w647 _]
              disable-tunnel: w591 -> [w604 w615 w627 w646 _]
              disable-tunnel: w589 -> [w608 w619 w631 w643 _]
              disable-tunnel: w588 -> [w606 w617 w629 w641 _]
              disable-tunnel: [w601 dbl[][] [] w628 w640 _] -> w576
              disable-tunnel: [w605 w616 w625 w639 _] -> w575
              frame Disabled {
                n236 = node "Python Node"(w609, w613, w608, w611, dbl[][] [], w606, w604) -> (w610:refnum<k35>, w612:errorcluster, w605:dbl[][])  [unwired: 2 in, 2 out]
                n237 = Array Subset(array=w604, index (row)=7 ("index"), length (row)=2 ("length")) -> (w601:dbl[][])  [unwired: 2 in]
              }
              frame Enabled {
                n238 = node "Python Node"(w620, w624, w619, w622, dbl[][] [], w617, w615) -> (w621:refnum<k35>, w623:errorcluster, w616:dbl[][])  [unwired: 2 in, 2 out]
              }
              frame Disabled {
                n239 = node "Python Node"(w634, w638, w631, w636, dbl[][] [], w629, w627) -> (w635:refnum<k35>, w637:errorcluster, w626:dbl[][])  [unwired: 2 in, 2 out]
                n240 = Delete From Array(array=w626, length=2, index (row)=5) -> (deleted portion=w628:dbl[][], array with subset deleted=w625:dbl[][])  [unwired: 1 in]
              }
              frame Disabled {
                n241 = Delete From Array(array=w646, length=2, index (row)=7) -> (deleted portion=w640:dbl[][], array with subset deleted=w652:dbl[][])  [unwired: 1 in]
                n242 = node "Python Node"(w647, w651, w643, w649, dbl[][] [], w641, w652) -> (w648:refnum<k35>, w650:errorcluster, w639:dbl[][])  [unwired: 2 in, 2 out]
              }
              frame Disabled {
              }
            }
            n243 = Close Python Session(session in=w593, error in=w595) -> (11:w580:errorcluster)
            n244 = Bundle By Name(cluster=w587, "XYZTheta Centers"=w575, "Pedestal Heights"=w576) -> (w583:T4)
            n245 = flat-sequence {
              tunnel: w583 -> [w661]
              tunnel: [w661] -> w586
              tunnel: w575 -> [w658]
              tunnel: w580 -> [w656]
              tunnel: [w655] -> w579
              tunnel: w586 -> [w663]
              tunnel: [w663] -> w585
              tunnel: [w662] -> w584
              tunnel: [w669] -> w582
              tunnel: w585 -> [w670]
              tunnel: w584 -> [w676]
              tunnel: w579 -> [w675]
              tunnel: [w674] -> w578
              tunnel: w577 -> [w673]
              tunnel: w576 -> [w672]
              tunnel: w575 -> [w671]
              frame #0 {
                n246 = local read "Position Number"() -> (w654:i16)
                n247 = call "even odd check.vi"("position"=w654) -> ("index"=w653:i32)  [unwired: 10 in]
                n248 = Index Array "Index Array"(array=w658, index (row)=w653) -> (element=w657:dbl[])  [unwired: 1 in]
                n249 = Reshape Array "Reshape Array"(w657, u32 4) -> (w660:dbl[])
                n250 = property on="Center" class="Arr (strict)"(error in=w656, "Val(Sgnl)"=w660) -> (error out=w655:errorcluster)  [unwired: 1 in, 1 out]
              }
              frame #1 {
                n251 = disable-structure shown="Enabled" {
                  disable-tunnel: [w664 TRUE ("T button?")] -> w662
                  frame Enabled {
                    n252 = Two Button Dialog(message="Ready to Submit?", 1:"No" ("F button name (\"Cancel\")"), 2:"Yes" ("T button name (\"OK\")")) -> (T button?=w664:bool)
                  }
                  frame Disabled {
                  }
                }
              }
              frame #2 {
                n253 = case shown="True" w676 {
                  tunnel: w675 -> [w678 w687]
                  tunnel: [w679 w686] -> w674
                  tunnel: w673 -> [_ w685]
                  tunnel: w672 -> [_ w684]
                  tunnel: w671 -> [_ w683]
                  tunnel: w670 -> [w677 w682]
                  tunnel: [w677 w681] -> w669
                  frame False {
                    n254 = property on="Enter Manual Mode" class="Bool (strict)"(error in=w678, "Val(Sgnl)"=TRUE ("Value (Signaling)")) -> (error out=w679:errorcluster)  [unwired: 1 in, 1 out]
                  }
                  frame True {
                    n255 = case shown="True" w685 {
                      selector: w685 -> [_ w696]
                      tunnel: w687 -> [w690 w698]
                      tunnel: [w689 w697] -> w686
                      tunnel: w684 -> [_ w695]
                      tunnel: w683 -> [_ w694]
                      tunnel: w682 -> [w688 w693]
                      tunnel: [w688 w692] -> w681
                      frame False {
                        n256 = property on="Auto Submit" class="Bool (strict)"(error in=w690, "Val(Sgnl)"=TRUE ("Value (Signaling)")) -> (error out=w689:errorcluster)  [unwired: 1 in, 1 out]
                      }
                      frame True {
                        n257 = disable-structure shown="Enabled" {
                          disable-tunnel: w698 -> [w710 w735]
                          disable-tunnel: [w709 w734] -> w697
                          disable-tunnel: w696 -> [w708 w733]
                          disable-tunnel: w695 -> [w707 _]
                          disable-tunnel: w694 -> [w706 _]
                          disable-tunnel: w693 -> [w701 w732]
                          disable-tunnel: [w700 w732] -> w692
                          frame Disabled {
                            n258 = disable-structure shown="Enabled" {
                              disable-tunnel: ["component thickness" 1.35 ("component thickness")] -> w702
                              frame Disabled {
                              }
                              frame Enabled {
                              }
                            }
                            n259 = property on="BP check" class="Bool (strict)"(error in=w710, "Val(Sgnl)"=w708) -> (error out=w709:errorcluster)  [unwired: 1 in, 1 out]
                            n260 = Array Subset(array=w706, index (row)=2 ("index"), length (row)=2 ("length")) -> (w703:dbl[][])  [unwired: 2 in]
                            n261 = for {
                              tunnel: w707 -> [w725] mode=indexing
                              tunnel: w703 -> [w723] mode=indexing
                              tunnel: w702 -> [w721]
                              tunnel: [w720] -> w699 mode=indexing
                              i -> [w717]
                              w719 = 2
                              n262 = Equal To 0?(x=w717) -> (x = 0?=w716:bool)
                              n263 = Index Array(array=w725, index=w719) -> (element=w724:dbl)
                              n264 = Select(t=0.5, s=w716, f=-0.5) -> (s? t:f=w713:dbl)
                              n265 = Add(x=w721, y=w724) -> (x+y=w722:dbl)
                              n266 = in-place {
                                in-place-border: w722 -> [w730]
                                in-place-border: w713 -> [w727]
                                n267 = in-place-array #3(w723, w719, 0) -> (w731:dbl, w728:dbl)
                                n268 = Subtract(x=w731, y=w730) -> (x-y=w729:dbl)
                                n269 = Add(x=w728, y=w727) -> (x+y=w726:dbl)
                                n270 = in-place-array #3(w729, w726) -> (w720:dbl[])  [unwired: 2 out]
                              }
                            }
                            n271 = Bundle By Name(cluster=w701, "Offset pins"=w699) -> (w700:T4)
                          }
                          frame Enabled {
                            n272 = property on="Auto Submit" class="Bool (strict)"(error in=w735, "Val(Sgnl)"=w733) -> (error out=w734:errorcluster)  [unwired: 1 in, 1 out]
                          }
                        }
                      }
                    }
                  }
                }
              }
            }
          }
        }
      }
      event "BP check": Value Change {
        n273 = event-data() -> ()  [unwired: 1 in, 6 out]
        n274 = flat-sequence {
          frame #0 {
            n275 = local write "Machine Vision"(Machine_Vision."None" ("Machine Vision")) -> ()
          }
          frame #1 {
            n276 = property on="BP check" class="Bool (strict)"("Value"=FALSE ("BP check")) -> ()  [unwired: 2 in, 2 out]
          }
        }
        n277 = Unbundle By Name(w759) -> ("XYZTheta Centers"=w773:dbl[][], "Offset pins"=w767:dbl[][])
        n278 = Array Subset(array=w773, index (row)=0 ("index"), length (row)=2 ("length")) -> (w770:dbl[][])  [unwired: 2 in]
        n279 = for {
          tunnel: w770 -> [w822] mode=indexing
          shift-right: [w806] -> w762
          shift-left: w769 -> [w787]
          shift-right: [w800] -> w766
          shift-left: w768 -> [w786]
          tunnel: w767 -> [w811] mode=indexing
          tunnel: [w799] -> w760 mode=indexing
          w797 = 300.0 ("Speed")
          n280 = Index Array(array=w811) -> (element #1=w816:dbl, element #2=w815:dbl, element #3=w798:dbl)  [unwired: 3 in]
          n281 = Build Array(w816, w815) -> (w814:dbl[])
          n282 = Replace Array Subset(array=w822, new element=w798, index=2) -> (w795:dbl[])
          n283 = Index Array(array=w795) -> (element #1=w793:dbl, element #2=w792:dbl, element #3=w790:dbl)  [unwired: 3 in]
          n284 = Build Array(w793, w792) -> (w791:dbl[])
          n285 = call "Z Go.vi"("Increment"=FALSE, "error in (no error)"=w786, "Speed In"=15.0, "Position In"=w790, "Gantry In"=w787) -> ("error out"=w785:errorcluster, "Gantry Out"=w784:refnum<k24>)  [unwired: 3 in, 2 out]
          n286 = call "XY Go.vi"("Increment?"=FALSE, "error in (no error)"=w785, "Speed"=w797, "XY In"=w791, "Gantry In"=w784) -> ("error out"=w782:errorcluster, "Gantry Out"=w783:refnum<k24>)  [unwired: 4 in, 1 out]
          n287 = call "Focus BP.vi"("error in"=w782, "Scan Inc"=0.01, "Start Inc"=-0.1, "Gantry In"=w783) -> ("error out"=w809:errorcluster, "max value"=w802:dbl, "Gantry Out"=w810:refnum<k24>)  [unwired: 5 in]
          n288 = call "XY Go.vi"("Increment?"=FALSE, "error in (no error)"=w809, "Speed"=w797, "XY In"=w814, "Gantry In"=w810) -> ("error out"=w818:errorcluster, "Gantry Out"=w819:refnum<k24>)  [unwired: 4 in, 1 out]
          n289 = call "Z Go.vi"("Increment"=FALSE, "error in (no error)"=w818, "Speed In"=15.0, "Position In"=w798, "Gantry In"=w819) -> ("error out"=w807:errorcluster, "Gantry Out"=w808:refnum<k24>)  [unwired: 3 in, 2 out]
          n290 = call "Focus BP.vi"("error in"=w807, "Scan Inc"=0.01, "Start Inc"=-0.1, "Gantry In"=w808) -> ("error out"=w800:errorcluster, "max value"=w801:dbl, "Gantry Out"=w806:refnum<k24>)  [unwired: 5 in]
          n291 = Subtract(x=w802, y=w801) -> (x-y=w805:dbl)
          n292 = Absolute Value(x=w805) -> (abs(x)=w804:dbl)
          n293 = Less?(x=w804, y=0.1) -> (x < y?=w799:bool)
        }
        n294 = And Array Elements(Boolean array=w760) -> (logical AND=w761:bool)
        n295 = case shown="True" w761 {
          selector: w761 -> [_ w781]
          tunnel: w766 -> [w776 w780]
          tunnel: [w775 w781] -> w765
          tunnel: [w774 w780] -> w764
          frame False {
            n296 = while {
              shift-right: [w778] -> w774
              shift-left: w776 -> [w779]
              tunnel: [w777] -> w775
              stop <- w777 stop-if-true
              n297 = call "Prompt User for Input2"("error in (no error)"=w779) -> ("Baseplate ready?"=w777:bool, "error out"=w778:errorcluster)  [unwired: 16 in, 1 out]
            }
          }
          frame True {
          }
        }
        n298 = property on="Auto Submit" class="Bool (strict)"(error in=w764, "Val(Sgnl)"=w765) -> (error out=w763:errorcluster)  [unwired: 1 in, 1 out]
      }
      event "Go to Center", "Position Number": Value Change {
        n299 = event-data() -> ()  [unwired: 1 in, 6 out]
        n300 = Unbundle By Name(w838) -> ("XYZTheta Centers"=w831:dbl[][])
        n301 = call "even odd check.vi"("position"="Position Number") -> ("index"=w827:i32)  [unwired: 10 in]
        n302 = Index Array "Index Array"(array=w831, index (row)=w827) -> (element=w833:dbl[])  [unwired: 1 in]
        n303 = Reshape Array "Reshape Array"(w833, u32 4) -> (w830:dbl[])
        n304 = case shown="True" "Go to Center" {
          tunnel: w830 -> [w839 w848]
          tunnel: w838 -> [w841 w850]
          tunnel: [w841 w850] -> w837
          tunnel: w835 -> [w840 w844]
          tunnel: [w840 w849] -> w832
          frame False {
            # "Change Position Number"
            "Center" <- w839
          }
          frame True {
            n305 = control-ref of="Joystick"() -> (w847:refnum<vi>)
            n306 = property class="Bool (strict)"(reference=w847) -> (reference out=w845:refnum<vi>, "Value"=w846:bool)  [unwired: 1 in, 1 out]
            n307 = case shown="True" w846 {
              selector: w846 -> [_ w856]
              tunnel: w844 -> [w851 w855]
              tunnel: [w851 w854] -> w843
              tunnel: w845 -> [_ w852]
              frame False {
              }
              frame True {
                n308 = Not(x=w856) -> (.not. x?=w853:bool)
                n309 = property class="Bool (strict)"(reference=w852, "Value"=w853) -> ()  [unwired: 1 in, 2 out]
                n310 = call "Joystick.vi"("Joystick"=w853, "Gantry In"=w855) -> ("Gantry Out"=w854:refnum<k24>)  [unwired: 8 in, 1 out]
              }
            }
            n311 = call "ClearXYZTheta Go.vi"("Speed"=300.0, "XYZTheta In"=w848, "Gantry In"=w843) -> ("Gantry Out"=w849:refnum<k24>)  [unwired: 6 in, 2 out]
          }
        }
      }
      event "Stop", "Auto Submit": Value Change {
        n312 = event-data() -> ()  [unwired: 1 in, 6 out]
        n313 = flat-sequence {
          frame #0 {
          }
          frame #1 {
            n314 = property on="Auto Submit" class="Bool (strict)"("Value"=FALSE ("Auto Submit")) -> ()  [unwired: 2 in, 2 out]
          }
        }
        n315 = property on="Both fiducials recorded" class="Bool (strict)"() -> ("Value"=w863:bool)  [unwired: 2 in, 2 out]
        n316 = property on="Stop" class="Bool"("DisabledEnum"=T7."Enabled" ("Disabled")) -> ()  [unwired: 2 in, 2 out]
        n317 = case shown="True" w863 {
          selector: w863 -> [w920 _]
          tunnel: [w920 w922] -> w858
          frame False {
            n318 = One Button Dialog(message="At least one fiducial not recorded!") -> ()  [unwired: 1 in, 1 out]
          }
          frame True {
            n319 = property on="Distance as expected?" class="Bool (strict)"() -> ("Value"=w923:bool)  [unwired: 2 in, 2 out]
            n320 = case shown="True" w923 {
              selector: w923 -> [w924 w926]
              tunnel: [w924 w926] -> w922
              frame False {
                n321 = One Button Dialog(message="Distance between fiducials does not match expected. Find fiducials again.") -> ()  [unwired: 1 in, 1 out]
              }
              frame True {
              }
            }
          }
        }
        "Program Done?" <- w858
        n322 = case shown="True" w858 {
          tunnel: w862 -> [w866 w898]
          tunnel: w861 -> [w867 w896]
          tunnel: [w867 w894] -> w860
          tunnel: [w866 w891] -> w859
          tunnel: w857 -> [_ w887]
          frame False {
          }
          frame True {
            n323 = Unbundle By Name(w887) -> ("Fiducials"=w886:path, "Gantry Fiducials"=w872:dbl[], "avg value count"=w881:dbl[], "Previous Avgs"=w885:dbl[][])
            n324 = call "Joystick.vi"("error in (no error)"=w898, "Joystick"=FALSE, "Gantry In"=w896) -> ("error out"=w899:errorcluster, "Gantry Out"=w894:refnum<k24>)  [unwired: 7 in]
            n325 = in-place {
              in-place-border: [w903] -> w880
              in-place-border: [w902] -> w879
              n326 = in-place-array #4(w881, 0) -> (w903:dbl)
              n327 = Increment(x=w903) -> (x+1=w902:dbl)
              n328 = in-place-array #4(w902) -> (w877:dbl[])  [unwired: 1 out]
            }
            n329 = Index Array(array=w872, index #1=2 ("index"), index #2=5 ("index")) -> (element #1=w869:dbl, element #2=w868:dbl)
            n330 = Multiply(x=w885, y=w880) -> (x*y=w890:dbl[][])
            n331 = Reshape Array(w872, 2 ("dimension size"), 3 ("dimension size")) -> (w882:dbl[][])
            n332 = for {
              tunnel: w882 -> [w907] mode=indexing
              tunnel: w890 -> [w908] mode=indexing
              tunnel: w879 -> [w905]
              tunnel: [w904] -> w889 mode=indexing
              n333 = Add(x=w907, y=w908) -> (x+y=w906:dbl[])
              n334 = Divide(x=w906, y=w905) -> (x/y=w904:dbl[])
            }
            n335 = Reshape Array(w889, 6 ("dimension size")) -> (w875:dbl[])
            n336 = in-place {
              in-place-border: w869 -> [w901]
              in-place-border: w868 -> [w900]
              n337 = in-place-array #5(w875, 2, 5) -> ()  [unwired: 2 out]
              n338 = in-place-array #5(w901, w900) -> (w873:dbl[])  [unwired: 2 out]
            }
            n339 = call "Replace Row In File.vi"("error in"=w899, "Index"=0, "Insert Array"=w873, "Path"=w886) -> ("error out"=w892:errorcluster)  [unwired: 7 in]
            n340 = call "Replace Row In File.vi"("error in"=w892, "Index"=1, "Insert Array"=w877, "Path"=w886) -> ("error out"=w891:errorcluster)  [unwired: 7 in]
          }
        }
        n341 = disable-structure shown="Enabled" {
          disable-tunnel: w859 -> [w910 w919]
          disable-tunnel: [_ w919] -> w865
          frame Disabled {
            n342 = case shown="No Error" w910 {
              tunnel: "Fiducial" -> [w911 w918]
              frame No Error {
                w912 = "\r"
                n343 = Concatenate Strings("Success!", w912, w912, w911, " Values Stored") -> ()  [unwired: 1 out]
              }
              frame Error {
                w915 = "\r"
                n344 = Concatenate Strings("Error!", w915, w915, w918, " Values Not Stored") -> ()  [unwired: 1 out]
              }
            }
          }
          frame Enabled {
          }
        }
      }
      event "Autofiducial (Beta)": Value Change {
        n345 = event-data() -> ()  [unwired: 1 in, 6 out]
        n346 = disable-structure shown="Enabled" {
          disable-tunnel: [w940 w973] -> w933
          disable-tunnel: w932 -> [w939 w973]
          disable-tunnel: "Autofiducial (Beta)" -> [w938 _]
          disable-tunnel: w929 -> [w936 _]
          disable-tunnel: [w934 _] -> w928
          frame Enabled {
            n347 = flat-sequence {
              tunnel: w938 -> [_]
              tunnel: [w946] -> w937
              tunnel: w939 -> [w951]
              tunnel: [w951] -> w945
              tunnel: [w950] -> w944
              tunnel: [w949] -> w943
              tunnel: w937 -> [w948]
              tunnel: w945 -> [w958]
              tunnel: [w957] -> w942
              tunnel: w944 -> [w956]
              tunnel: [w955] -> w941
              tunnel: w943 -> [w955]
              tunnel: w936 -> [w954]
              tunnel: [w952] -> w935
              tunnel: [w967] -> w940
              tunnel: w942 -> [w968]
              tunnel: w941 -> [w966]
              tunnel: w935 -> [w965]
              tunnel: [w963] -> w934
              frame #0 {
                n348 = local read "Image"() -> (w947:T5)
                n349 = call "Find Fiducial.vi"("Image"=w947) -> ("Move by (mm)"=w946:dbl[])  [unwired: 3 in]
              }
              frame #1 {
                n350 = Index Array(array=w948) -> (element #1=w950:dbl, element #2=w949:dbl)  [unwired: 2 in]
                "Move by" <- w948
              }
              frame #2 {
                n351 = call "Joystick.vi"("error in (no error)"=w954, "Joystick"=FALSE, "Gantry In"=w958) -> ("error out"=w953:errorcluster, "Gantry Out"=w959:refnum<k24>)  [unwired: 7 in]
                n352 = call "Move Inc.vi"("Axis"="X", "error in (no error)"=w953, "Speed"=25.0, "Distance"=w956, "Gantry In"=w959) -> ("error out"=w952:errorcluster, "Gantry Out"=w957:refnum<k24>)  [unwired: 5 in]
              }
              frame #3 {
                n353 = call "Joystick.vi"("error in (no error)"=w965, "Joystick"=FALSE, "Gantry In"=w968) -> ("error out"=w964:errorcluster, "Gantry Out"=w969:refnum<k24>)  [unwired: 7 in]
                n354 = call "Move Inc.vi"("Axis"="Y", "error in (no error)"=w964, "Speed"=25.0, "Distance"=w966, "Gantry In"=w969) -> ("error out"=w963:errorcluster, "Gantry Out"=w967:refnum<k24>)  [unwired: 5 in]
              }
            }
          }
          frame Disabled {
          }
        }
      }
    }
    n355 = Equal?(x=w94, y=0) -> (x = y?=w92:bool)
    n356 = case shown="True" w92 {
      selector: w92 -> [_ w108]
      tunnel: w91 -> [_ w103]
      frame False {
      }
      frame True {
        w107 = T7."Disabled and Grayed Out" ("Disabled")
        n357 = property on="Go to Top Left Fiducial" class="Bool (strict)"("Val(Sgnl)"=w108) -> ()  [unwired: 2 in, 2 out]
        n358 = Unbundle By Name(w103) -> ("Assembly Type"=w102:string, "Tray Number"=w100:string)  [unwired: 1 out]
        n359 = property on="Stop" class="Bool"("DisabledEnum"=w107) -> ()  [unwired: 2 in, 2 out]
        n360 = Concatenate Strings("Now measuring Tray " ("initial string"), w100, " for " ("string"), w102) -> (→"resulting string":string)
        n361 = property on="Go to Center" class="Bool"("DisabledEnum"=w107) -> ()  [unwired: 2 in, 2 out]
        n362 = property on="Record Top Right" class="Bool (strict)"("DisabledEnum"=w107) -> ()  [unwired: 2 in, 2 out]
        n363 = property on="Go to Top Right Fiducial" class="Bool (strict)"("DisabledEnum"=w107) -> ()  [unwired: 2 in, 2 out]
        n364 = property on="Record Top Left" class="Bool (strict)"("DisabledEnum"=w107) -> ()  [unwired: 2 in, 2 out]
        n365 = property on="Go to Top Left Fiducial" class="Bool (strict)"("DisabledEnum"=w107) -> ()  [unwired: 2 in, 2 out]
        "Instructions" <- "Answer prompts then wait for gantry movement." ("Instructions")
      }
    }
  }
  "Gantry Out" <- w11
  "error out" <- w3
  n366 = Unbundle By Name(w13) -> ("XYZTheta Centers"=→"XYZTheta Centers":dbl[][], "Pedestal Heights"=→"Pedestal Heights":dbl[][])
